vi "ZCAN_FilterSheet(DTU).vi"(0 "error in (no error)":errorcluster caption="错误输入（无错误）", 2 "can_index_handle":u32, 5 "can_index":u32, 9 "acc_code":string, 11 "acc_mask":string) -> (14 "error out":errorcluster caption="错误输出", 15 "success?":bool, 16 "can_index_handle（out）":u32, 19 "can_index (out)":u32)   [LabVIEW 2018]
doc: "设置滤波表格"
uses:
  zlgcan_demo_CANFDNET_UDP/bin/zlgcan_wrap.dll
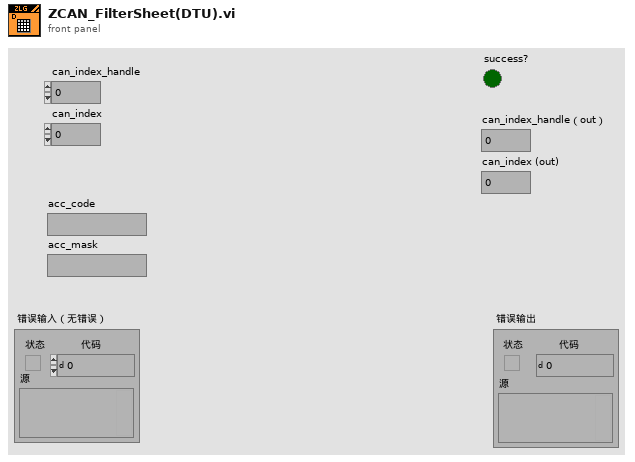
[diagram p1: front panel]
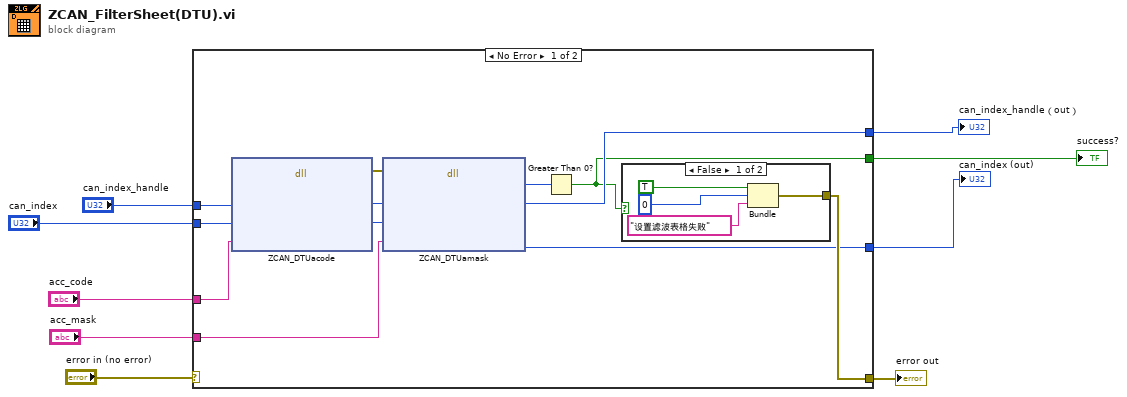
[diagram p0: block diagram]
diagram:
  n1 = case shown="No Error" "error in (no error)" {
    selector: "error in (no error)" -> [_ w26]
    tunnel: [w15 w26] -> w8
    tunnel: "can_index_handle" -> [w18 _]
    tunnel: "can_index" -> [w17 _]
    tunnel: "acc_code" -> [w14 _]
    tunnel: "acc_mask" -> [w13 _]
    tunnel: [w12 _] -> w3
    tunnel: [w11 _] -> w2
    tunnel: [w10 _] -> w1
    frame No Error {
      n2 = dll-call lib="C:/Users/admin/Desktop/zlgcan_demo_CANFDNET_UDP/bin/zlgcan_wrap.dll" fn="ZCAN_DTUacode"("device_handle"=w18, "can_index"=w17, "acc_code"=w14) -> (error out=w21:errorcluster, "device_handle"=w19:u32, "can_index"=w20:u32)  [unwired: 5 in, 1 out]
      n3 = dll-call lib="C:/Users/admin/Desktop/zlgcan_demo_CANFDNET_UDP/bin/zlgcan_wrap.dll" fn="ZCAN_DTUamask"(error in=w21, "device_handle"=w19, "can_index"=w20, "acc_mask"=w13) -> ("return"=w16:u32, "device_handle"=w12:u32, "can_index"=w11:u32)  [unwired: 3 in, 2 out]
      n4 = Greater Than 0?(x=w16) -> (x > 0?=w10:bool)
      n5 = case shown="False" w10 {
        tunnel: [w22 _] -> w15
        frame False {
          n6 = Bundle("status"=TRUE, "code"=0, "消息"="设置滤波表格失败") -> (w22:cluster{"status":bool, "code":i32, "消息":string})  [unwired: 1 in]
        }
        frame True {
        }
      }
    }
    frame Error {
    }
  }
  "error out" <- w8
  "can_index_handle（out）" <- w3
  "can_index (out)" <- w2
  "success?" <- w1
